vi "SerialWhere.vi"(2 "error in (no error)":errorcluster, 4 "Axis":string) -> (0 "error out":errorcluster, 1 "Output":dbl format="%#.1f")   [LabVIEW 2010]
doc: "Establishes connection with configured port (default = COM1).\nSends command MOVE X=x Y=y where x and y are integers denoting 10ths of a micron.\nSub-VI SerialWaitForStatusN.vi polls controller with STATUS command until 'N' (not busy) status is returned, or until a configured maximum number of unsuccessful tries (default = 400).\nDisconnects from configured port."
uses:
  <vilib>/Instr/_visa.llb/VISA Configure Serial Port (Instr).vi
panel:
  in  "timeout (10sec)":u32=100
  # "Note: This VI ships with 100 ms as the default timeout value. That means that the\nVI will listen to the MS2000 for up to 100 ms after sending a command.\nMS2000 terminates its reply with CR. This VI is configured by VISA Configure Serial Port.vi\nto stop listening when it receives a CR (decimal 13). \nNormally the MS2000 completes its reply within the 100 ms timeout. This timeout value\ncan be adjusted down for faster performance.\nHowever, if too low, then the VI may not wait long enough for the MS2000\nto reply to the command."
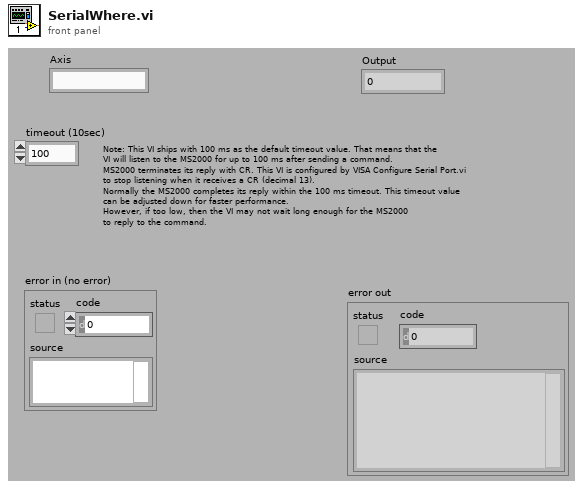
[diagram p1: front panel]
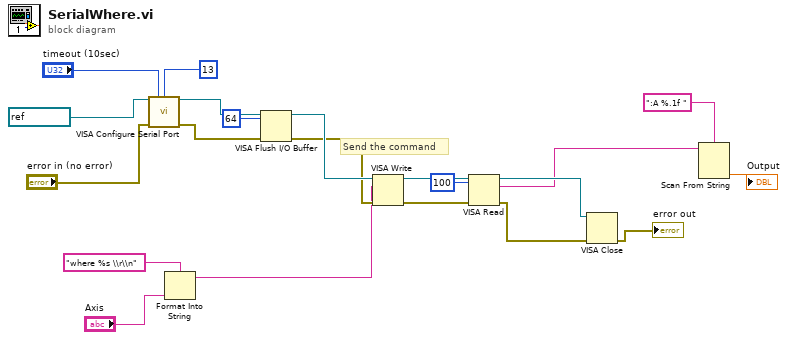
[diagram p0: block diagram]
diagram:
  # "Send the command"
  n1 = call-poly "VISA Configure Serial Port"("VISA resource name"=refnum<visa-resource-name> "COM3", "timeout (10sec)"="timeout (10sec)", "termination char\n(0xA = '\\n' = LF)"=u8 13 ("termination char\n(0xA = '\\n' = LF)"), "error in (no error)"="error in (no error)") -> ("VISA resource name out"=w16:refnum<visa-resource-name>, "error out"=w14:errorcluster)  [unwired: 10 in]
  n2 = Format Into String "Format Into String"(format string="where %s \\r\\n", "Axis") -> (resulting string=w1:string)  [unwired: 2 in, 1 out]
  n3 = VISA Flush I/O Buffer(VISA resource name=w16, mask (16)=u16 64, error in (no error)=w14) -> (VISA resource name out=w19:refnum<visa-resource-name>, error out=w18:errorcluster)
  n4 = VISA Write(VISA resource name=w19, write buffer=w1, error in (no error)=w18) -> (VISA resource name out=w21:refnum<visa-resource-name>, error out=w9:errorcluster)  [unwired: 1 out]
  n5 = VISA Read(VISA resource name=w21, byte count=u32 100, error in (no error)=w9) -> (VISA resource name out=w10:refnum<visa-resource-name>, read buffer=w4:string, error out=w11:errorcluster)  [unwired: 1 out]
  n6 = VISA Close(VISA resource name=w10, error in (no error)=w11) -> (error out=→"error out":errorcluster)
  n7 = Scan From String "Scan From String"(format string=":A %.1f ", input string=w4) -> (output 1=→"Output":dbl)  [unwired: 3 in, 3 out]
